vi "test_5782_stage1.vi"() -> ()   [LabVIEW 2013]
uses:
  <vilib>/measure/maspectr.llb/Power Spectrum and PSD Export Mode.ctl
  <vilib>/measure/maspectr.llb/FFT Power Spectrum and PSD for 1 Chan (CDB).vi
  <vilib>/measure/NI_MAPro.lvlib
panel:
  out "Waveform Graph 3":dbl[](graph)
  out "min value":i16
  out "max value":i16
  out "Waveform Graph 2":i16[](graph)
  out "size before":i32
  out "Waveform Graph":dbl[][](graph)
  out "power spectrum":cluster{"f0":dbl, "df":dbl, "magnitude":dbl[]}(graph)
  out "size after":i32
  out "Q out":fxp<+/-,16,14>[](array[numeric])
  out "I out":fxp<+/-,16,14>[](array[numeric])
  out "iteration1":i32
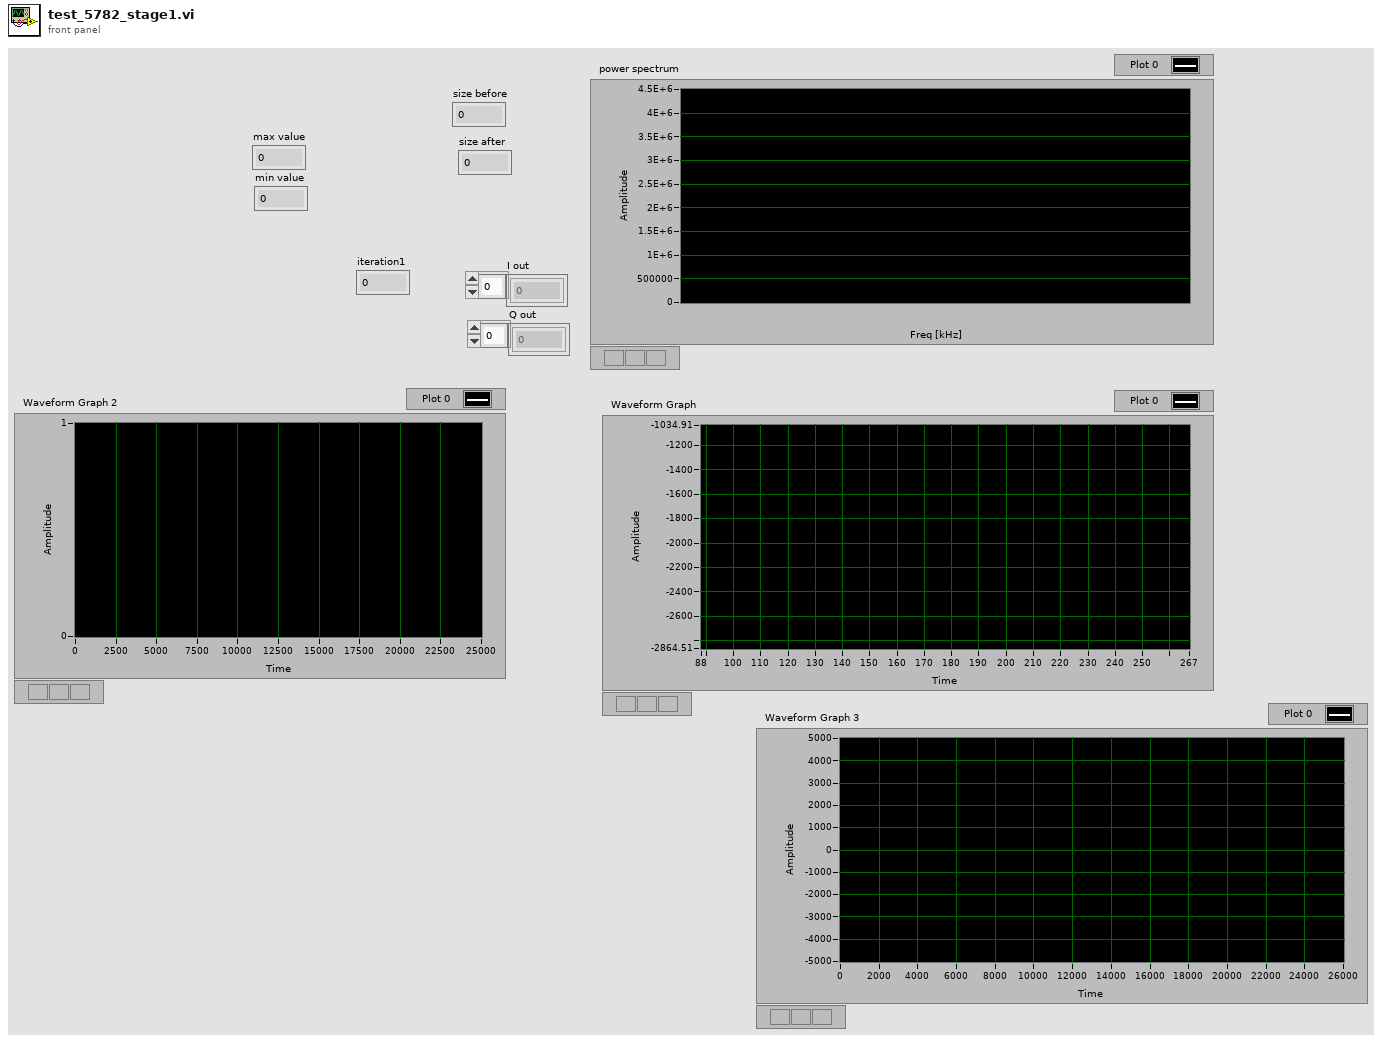
[diagram p1: front panel]
types:
  T1 = typedef "NI_MAPro.lvlib/Power Spectrum and PSD Export Mode.ctl" = u16
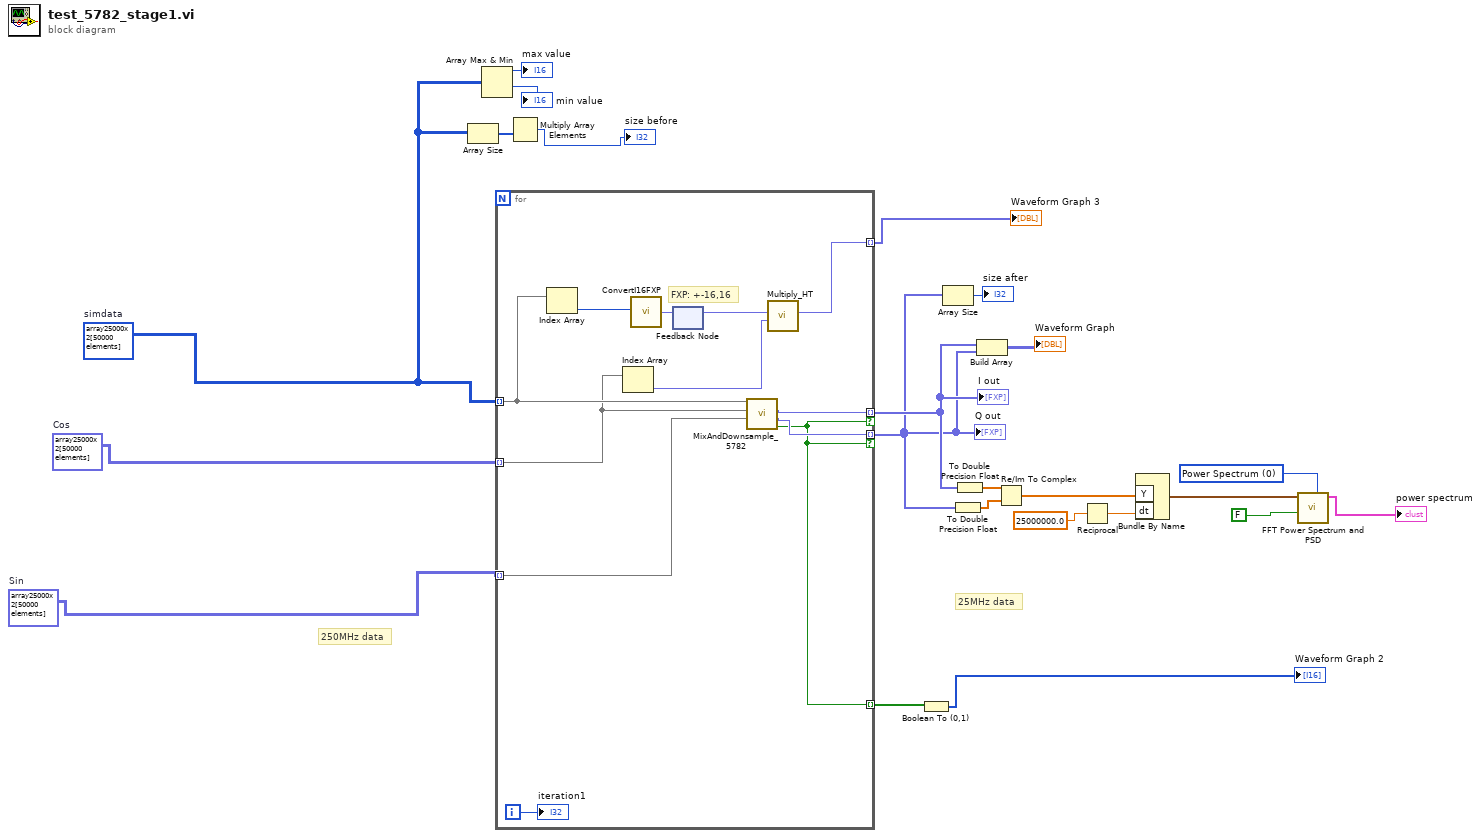
[diagram p0: block diagram]
diagram:
  w3 = fxp<+/-,16,0>[][] array25000x2[50000 elements]  # Cos
  w1 = i16[][] array25000x2[50000 elements]  # simdata
  w2 = fxp<+/-,16,0>[][] array25000x2[50000 elements]  # Sin
  w22 = T1 0 items=["Power Spectrum", "Power Spectral Density"] ("export mode")
  # "25MHz data"
  # "250MHz data"
  n1 = Array Size(array=w1) -> (size(s)=w13:i32[])
  n2 = Array Max & Min(array=w1) -> (max value=→"max value":i16, min value=→"min value":i16)  [unwired: 2 out]
  n3 = for {
    tunnel: [w33] -> w9 mode=indexing if=w31
    tunnel: [w32] -> w8 mode=indexing if=w31
    tunnel: w1 -> [w28] mode=indexing
    tunnel: w2 -> [w34] mode=indexing
    tunnel: w3 -> [w26] mode=indexing
    tunnel: [w31] -> w11 mode=indexing
    tunnel: [w24] -> w4 mode=indexing
    i -> [w35]
    # "FXP: +-16,16"
    n4 = Index Array(array=w28) -> (element=w27:i16)  [unwired: 1 in]
    n5 = Index Array(array=w26) -> (element=w25:fxp<+/-,16,0>)  [unwired: 1 in]
    n6 = call "ConvertI16FXP.vi"("I16"=w27) -> ("y"=w30:fxp<+/-,16,16>)
    n7 = feedback #1() -> (w29:fxp<+/-,16,16>)  [unwired: 1 in]
    n8 = feedback-in #1(w30) -> ()
    n9 = call "MixAndDownsample_5782.vi"("Sine in"=w34, "Cosine in"=w26, "Signal Input"=w28) -> ("data valid"=w31:bool, "Q out"=w32:fxp<+/-,16,14>, "I out"=w33:fxp<+/-,16,14>)  [unwired: 6 in]
    n10 = call "Multiply_HT.vi"("DDS sample"=w25, "Signal sample"=w29) -> ("Output"=w24:fxp<+/-,16,14>)  [unwired: 8 in, 1 out]
    "iteration1" <- w35
  }
  "I out" <- w9
  "Q out" <- w8
  "Waveform Graph 3" <- w4
  n11 = Multiply Array Elements(1:w13) -> (0:→"size before":i32)
  n12 = Boolean To (0,1)(Boolean=w11) -> (0, 1=→"Waveform Graph 2":i16[])
  n13 = Array Size(array=w8) -> (size(s)=→"size after":i32)
  n14 = To Double Precision Float(number=w8) -> (double precision float=w15:dbl[])
  n15 = To Double Precision Float(number=w9) -> (double precision float=w16:dbl[])
  n16 = Build Array(w9, w8) -> (→"Waveform Graph":fxp<+/-,16,14>[][])
  n17 = Re/Im To Complex(1:w15, 2:w16) -> (0:w14:cdb[])
  n18 = Reciprocal(x=25000000.0 ("dt")) -> (1/x=w18:dbl)
  n19 = Bundle By Name("Y"=w14, "dt"=w18) -> (w21:waveform(cdb))  [unwired: 1 in]
  n20 = call-poly <vilib>:"FFT Power Spectrum and PSD.vi"("export mode"=w22, "dB On (F)"=FALSE, "time signal"=w21) -> ("Power Spectrum / PSD"=→"power spectrum":cluster{"f0":dbl, "df":dbl, "magnitude":dbl[]})  [unwired: 5 in, 3 out]
